vi "_DeviceAttributesList.vi"(0 "device name":string) -> (1 "error stack":string[](array[string]), 2 "attributes_list":string[](array[string]), 3 "success":bool=TRUE)   [LabVIEW 2014, in "tango.lvlib"]
uses:
  tango.lvlib
  tango_binding.so
panel:
  # "This Vi is deprecated and only maintained for backward compatibility. Please use  _TangoAttributesList instead."
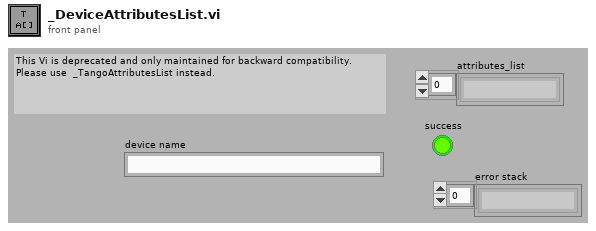
[diagram p1: front panel]
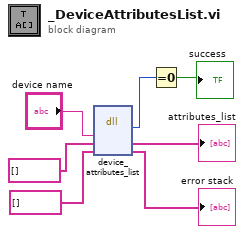
[diagram p0: block diagram]
diagram:
  n1 = dll-call lib="tango_binding.*" fn="device_attributes_list"("dev_name"="device name", "attributes_list"=string[] [] ("Error Stack"), "error_stack"=string[] [] ("Error Stack")) -> ("return type"=w5:i32, "attributes_list"=→"attributes_list":string[], "error_stack"=→"error stack":string[])  [unwired: 4 in, 2 out]
  n2 = Equal To 0?(x=w5) -> (x = 0?=→"success":bool)
